vi "SubVI_Prescan marker.vi"(5 "corrected 2D array":dbl[][](array[numeric]), 6 "Column to Sort on":i32=1, 7 "corrected amplitude 1D arrray":dbl[](array[numeric]), 9 "limit 1D array":dbl[](array[numeric]), 10 "frequency 1D array":dbl[](array[numeric])) -> (1 "corrected 2D array\nwith limit and margin":dbl[][](array[numeric]), 2 "sorted array":dbl[][](array[numeric]), 4 "6 entries in table":dbl[][](array[numeric]))   [LabVIEW 2016]
panel:
  out "subarray 3":dbl[](array[numeric])
  out "subarray 4":dbl[](array[numeric])
  out "subarray 5":dbl[](array[numeric])
  out "subarray 2":dbl[](array[numeric])
  out "subarray 1":dbl[](array[numeric])
  out "subarray 0":dbl[](array[numeric])
  out "x-y":dbl[](array[numeric])
  out "limit":dbl[](array[numeric])
  out "XY Graph":T1(graph)
  out "value":dbl[](array[numeric])
  out "X-axis":dbl[](array[numeric])
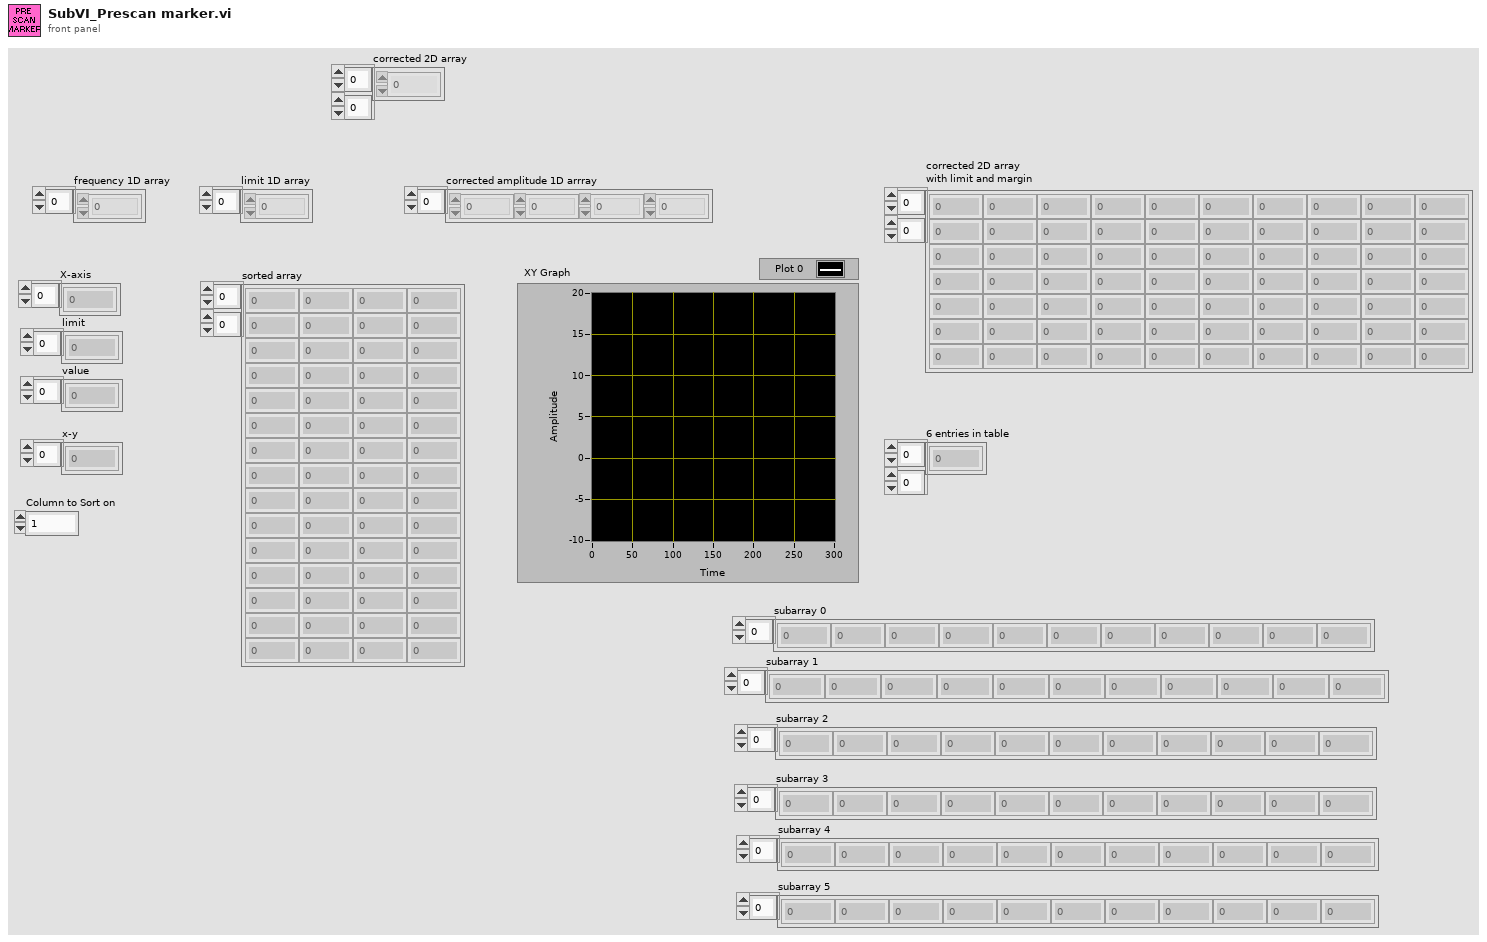
[diagram p1: front panel]
types:
  T1 = cluster{"frequency 1D array":dbl[], "limit 1D array":dbl[]}[]
  T2 = cluster{"frequency 1D array":dbl[], "corrected amplitude 1D arrray":dbl[]}
  T3 = cluster{"frequency 1D array":dbl[], "limit 1D array":dbl[]}
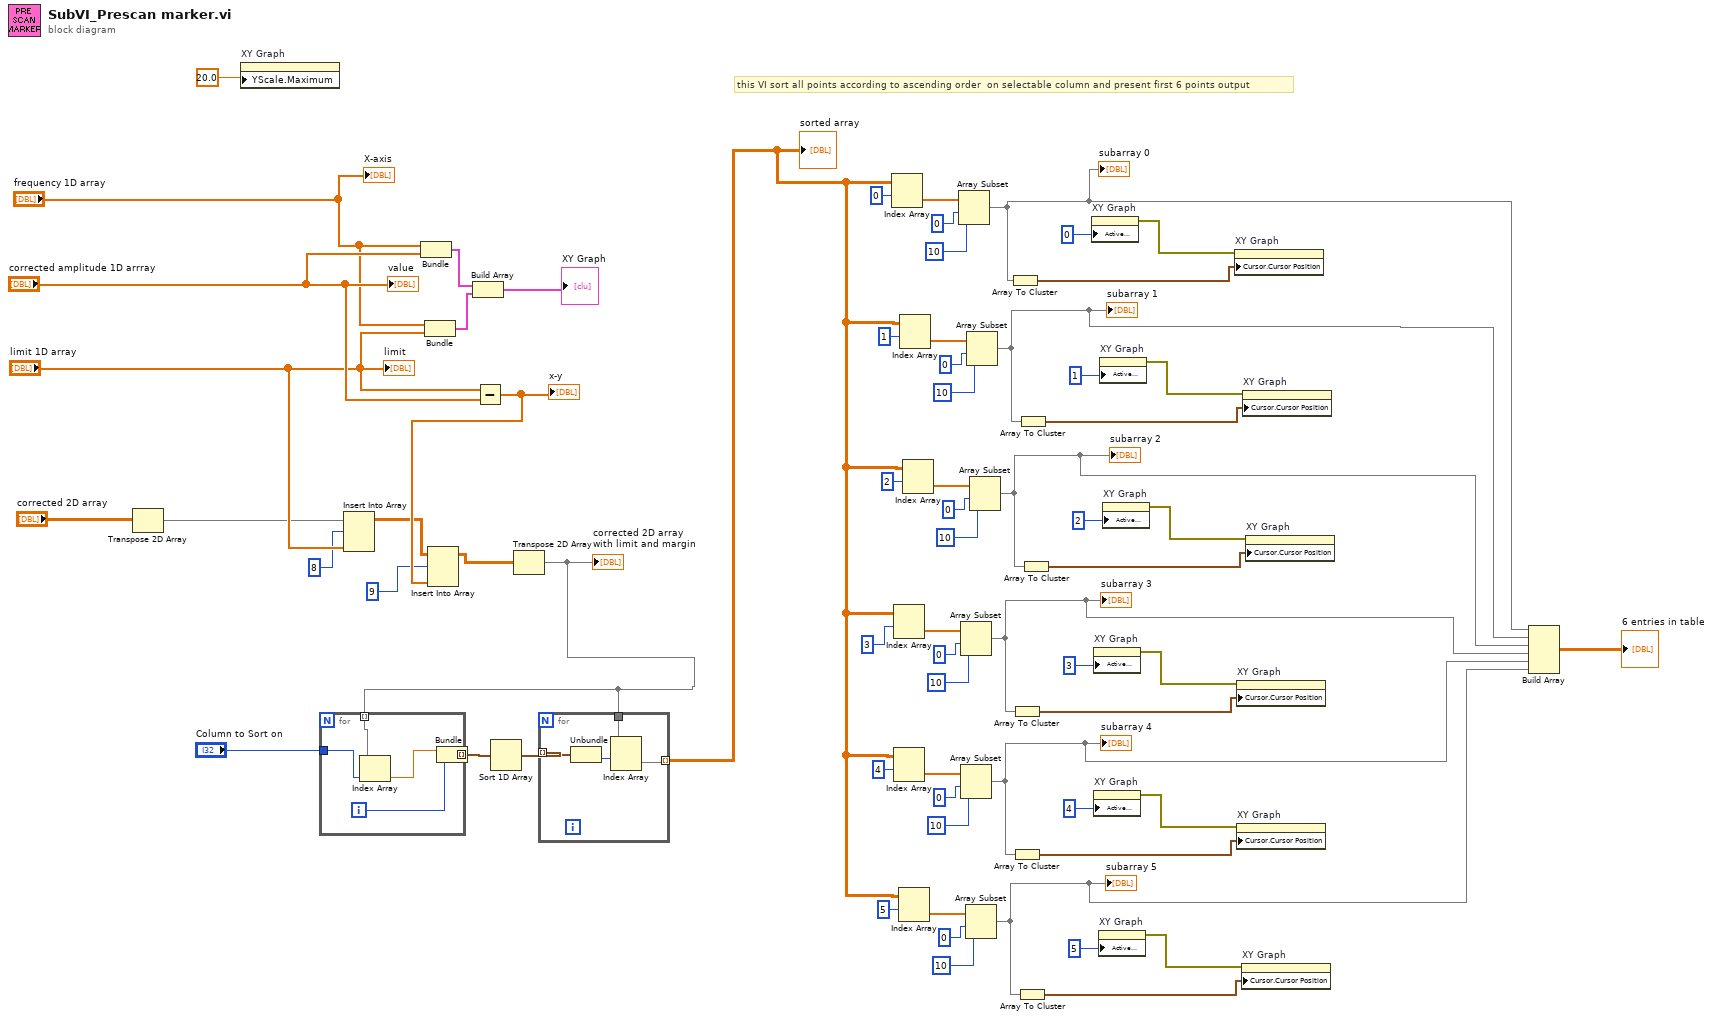
[diagram p0: block diagram]
diagram:
  # "this VI sort all points according to ascending order  on selectable column and present first 6 points output"
  n1 = Transpose 2D Array(2D array="corrected 2D array") -> (transposed array=w12:dbl[][])
  n2 = property on="XY Graph" class="XYGraph (strict)"("YScale.Maximum"=20.0 ("Y Scale.Range:Maximum")) -> ()  [unwired: 2 in, 2 out]
  n3 = Insert Into Array(array=w12, index (row)=8, new element="limit 1D array") -> (w14:dbl[][])  [unwired: 1 in]
  n4 = Bundle("frequency 1D array"="frequency 1D array", "corrected amplitude 1D arrray"="corrected amplitude 1D arrray") -> (w68:T2)  [unwired: 1 in]
  n5 = Bundle("frequency 1D array"="frequency 1D array", "limit 1D array"="limit 1D array") -> (w67:T3)  [unwired: 1 in]
  n6 = Build Array(w68, w67) -> (→"XY Graph":T1)
  n7 = Subtract(x="limit 1D array", y="corrected amplitude 1D arrray") -> (x-y=w15:dbl[])
  "x-y" <- w15
  n8 = Insert Into Array(array=w14, index (row)=9, new element=w15) -> (w11:dbl[][])  [unwired: 1 in]
  n9 = Transpose 2D Array(2D array=w11) -> (transposed array=w8:dbl[][])
  "corrected 2D array\nwith limit and margin" <- w8
  n10 = for {
    tunnel: w8 -> [w69] mode=indexing
    tunnel: [w71] -> w63 mode=indexing
    tunnel: "Column to Sort on" -> [w73]
    i -> [w72]
    n11 = Index Array(array=w69, index=w73) -> (element=w70:dbl)
    n12 = Bundle(w70, w72) -> (w71:cluster{dbl, i32})  [unwired: 1 in]
  }
  n13 = Sort 1D Array(array=w63) -> (sorted array=w62:cluster{dbl, i32}[])
  n14 = for {
    tunnel: w62 -> [w77] mode=indexing
    tunnel: [w75] -> w19 mode=indexing
    tunnel: w8 -> [w76]
    n15 = Unbundle(w77) -> (w74:i32)  [unwired: 1 out]
    n16 = Index Array(array=w76, index (row)=w74) -> (element=w75:dbl[])  [unwired: 1 in]
  }
  "sorted array" <- w19
  n17 = Index Array(array=w19, index (row)=0) -> (element=w58:dbl[])  [unwired: 1 in]
  n18 = Index Array(array=w19, index (row)=3) -> (element=w23:dbl[])  [unwired: 1 in]
  n19 = Index Array(array=w19, index (row)=4) -> (element=w30:dbl[])  [unwired: 1 in]
  n20 = Index Array(array=w19, index (row)=5) -> (element=w37:dbl[])  [unwired: 1 in]
  n21 = Index Array(array=w19, index (row)=1) -> (element=w51:dbl[])  [unwired: 1 in]
  n22 = Index Array(array=w19, index (row)=2) -> (element=w44:dbl[])  [unwired: 1 in]
  n23 = Array Subset(array=w58, index=0, length=10) -> (w7:dbl[])
  "subarray 0" <- w7
  n24 = Array Subset(array=w23, index=0, length=10) -> (w4:dbl[])
  "subarray 3" <- w4
  n25 = Array Subset(array=w30, index=0, length=10) -> (w3:dbl[])
  "subarray 4" <- w3
  n26 = Array Subset(array=w37, index=0, length=10) -> (w2:dbl[])
  "subarray 5" <- w2
  n27 = Array Subset(array=w51, index=0, length=10) -> (w6:dbl[])
  "subarray 1" <- w6
  n28 = Array Subset(array=w44, index=0, length=10) -> (w5:dbl[])
  "subarray 2" <- w5
  n29 = Array To Cluster(array=w7) -> (cluster=w55:cluster{"[0]":dbl, "[1]":dbl})
  n30 = Array To Cluster(array=w4) -> (cluster=w26:cluster{"[0]":dbl, "[1]":dbl})
  n31 = Array To Cluster(array=w3) -> (cluster=w27:cluster{"[0]":dbl, "[1]":dbl})
  n32 = Array To Cluster(array=w2) -> (cluster=w40:cluster{"[0]":dbl, "[1]":dbl})
  n33 = Array To Cluster(array=w6) -> (cluster=w54:cluster{"[0]":dbl, "[1]":dbl})
  n34 = Array To Cluster(array=w5) -> (cluster=w41:cluster{"[0]":dbl, "[1]":dbl})
  n35 = property on="XY Graph" class="XYGraph (strict)"("Active Cursor"=u32 0) -> (error out=w61:errorcluster)  [unwired: 2 in, 1 out]
  n36 = property on="XY Graph" class="XYGraph (strict)"("Active Cursor"=u32 3) -> (error out=w20:errorcluster)  [unwired: 2 in, 1 out]
  n37 = property on="XY Graph" class="XYGraph (strict)"("Active Cursor"=u32 4) -> (error out=w33:errorcluster)  [unwired: 2 in, 1 out]
  n38 = property on="XY Graph" class="XYGraph (strict)"("Active Cursor"=u32 5) -> (error out=w34:errorcluster)  [unwired: 2 in, 1 out]
  n39 = property on="XY Graph" class="XYGraph (strict)"("Active Cursor"=u32 1) -> (error out=w48:errorcluster)  [unwired: 2 in, 1 out]
  n40 = property on="XY Graph" class="XYGraph (strict)"("Active Cursor"=u32 2) -> (error out=w47:errorcluster)  [unwired: 2 in, 1 out]
  n41 = property on="XY Graph" class="XYGraph (strict)"(error in=w61, "Cursor.Cursor Position"=w55) -> ()  [unwired: 1 in, 2 out]
  n42 = property on="XY Graph" class="XYGraph (strict)"(error in=w20, "Cursor.Cursor Position"=w26) -> ()  [unwired: 1 in, 2 out]
  n43 = property on="XY Graph" class="XYGraph (strict)"(error in=w33, "Cursor.Cursor Position"=w27) -> ()  [unwired: 1 in, 2 out]
  n44 = property on="XY Graph" class="XYGraph (strict)"(error in=w34, "Cursor.Cursor Position"=w40) -> ()  [unwired: 1 in, 2 out]
  n45 = property on="XY Graph" class="XYGraph (strict)"(error in=w48, "Cursor.Cursor Position"=w54) -> ()  [unwired: 1 in, 2 out]
  n46 = property on="XY Graph" class="XYGraph (strict)"(error in=w47, "Cursor.Cursor Position"=w41) -> ()  [unwired: 1 in, 2 out]
  n47 = Build Array(w7, w6, w5, w4, w3, w2) -> (→"6 entries in table":dbl[][])
  "X-axis" <- "frequency 1D array"
  "value" <- "corrected amplitude 1D arrray"
  "limit" <- "limit 1D array"
